vi "Write SA Pin.vi"(8 "error in (no error)":errorcluster, 10 "SA Pin":string, 11 "LTE_SEM in":refnum<class "LTE_SEM.lvclass">=refnum) -> (0 "error out":errorcluster, 3 "LTE_SEM out":refnum<class "LTE_SEM.lvclass">)   [LabVIEW 2016, in "SeqAuto Evaluations.lvlib" / "LTE_SEM.lvclass"]
uses:
  LTE_SEM.lvclass
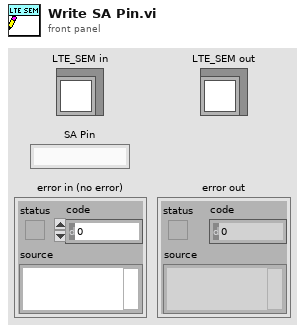
[diagram p1: front panel]
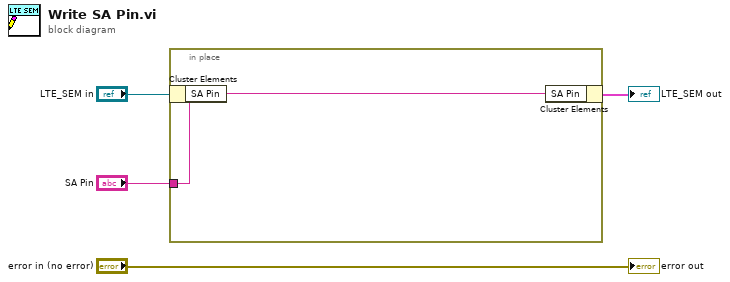
[diagram p0: block diagram]
diagram:
  n1 = in-place {
    in-place-border: "SA Pin" -> [w5]
    n2 = in-place-cluster #1("LTE_SEM in") -> ()  [unwired: 1 out]
    n3 = in-place-cluster #1("SA Pin"=w5) -> (→"LTE_SEM out":cluster{})
  }
  "error out" <- "error in (no error)"
